vi "Set picture background.vi"(8 "error in":errorcluster, 9 "pic height":i16, 10 "pic width":i16, 11 "Theme in":refnum<class "Theme.lvclass">) -> (0 "error out":errorcluster, 2 "background":picture, 3 "Theme out":refnum<class "Theme.lvclass">)   [LabVIEW 2021, in "Theme.lvclass"]
doc: "Set the background of a picture to the specified color\n\n<b>Code Developed By:</b> +\nDaniel Coons +\nhttps://github.com/danielcoons/tsc-pop-up"
uses:
  Theme.lvclass
  Theme.lvclass/Theme.ctl
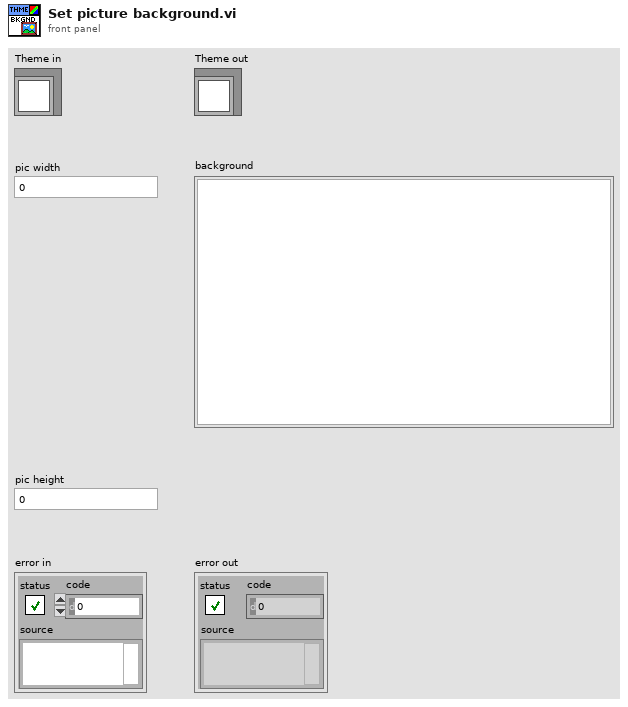
[diagram p1: front panel]
types:
  T1 = cluster{"left":i16, "top":i16, "right":i16, "bottom":i16}
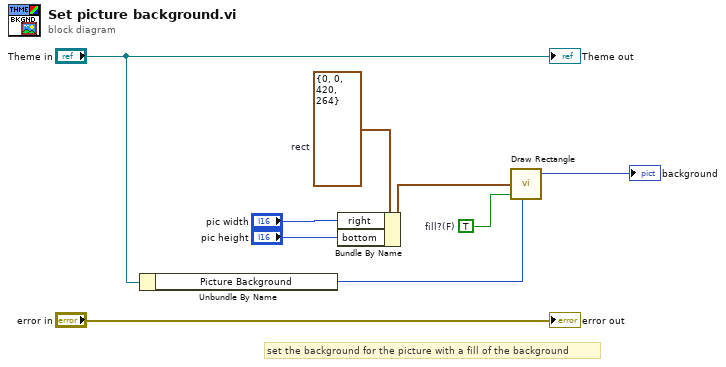
[diagram p0: block diagram]
diagram:
  w2 = T1 {"left"=0, "top"=0, "right"=420, "bottom"=264}  # rect
  w8 = TRUE  # fill?(F)
  # "set the background for the picture with a fill of the background"
  n1 = Unbundle By Name("Theme in") -> ("Picture Background"=w5:u32)
  n2 = Bundle By Name(cluster=w2, "right"="pic width", "bottom"="pic height") -> (w1:T1)
  n3 = call <vilib>:"Draw Rectangle.vi"("rect"=w1, "fill?(F)"=w8, "color(black)"=w5) -> ("new picture"=→"background":picture)  [unwired: 6 in]
  "error out" <- "error in"
  "Theme out" <- "Theme in"
